vi "IMUCompute.vi"(10 "Cluster":T16 {"navX Device TypeDef"."navX Common Information"."Update Rate (4Hz-60Hz)" min=4 max=50 step=1; "navX Device TypeDef"."navX System Information"."Status"."NAVX_OP_STATUS" items=["INITIALIZING", "SELFTEST_IN_PROGRESS", "ERROR", "IMU_AUTOCAL_IN_PROGRESS", "NORMAL"]; "navX Device TypeDef"."navX System Information"."Status"."NAVX_CAL_STATUS" items=["IMU_CAL_STATE_MASK"=3, "IMU_CAL_INPROGRESS"=0, "IMU_CAL_ACCUMULATE"=1, "IMU_CAL_COMPLETE"=2, "MAG_CAL_COMPLETE"=4, "BARO_CAL_COMPLETE"=8]; "navX Device TypeDef"."navX Interface Protocol TypeDefs"."I2CDevRef"."Device Address" format="%.0x"}) -> ()   [LabVIEW 2014]
uses:
  NavX/roborio/labview/navX-MXP Library/COMMON/TypeDefs/Data TypeDefs/navX Vector Data.ctl
  NavX/roborio/labview/navX-MXP Library/COMMON/TypeDefs/navX Device TypeDef.ctl
  NavX/roborio/labview/navX-MXP Library/COMMON/TypeDefs/Value TypeDefs/navX Interface Protocol.ctl
  <vilib>/Rock Robotics/WPI/SPI/WPI_SPIDevRef.ctl
  <vilib>/Rock Robotics/SystemInterfaces/Typedef/FPGA_TypedefDigitalModule.ctl
  <vilib>/Rock Robotics/SystemInterfaces/spilib/spi_bus.ctl
  <vilib>/Rock Robotics/WPI/I2C/WPI_I2CDevRef.ctl
  <vilib>/Rock Robotics/SystemInterfaces/i2clib/i2c_bus.ctl
  NavX/roborio/labview/navX-MXP Library/COMMON/TypeDefs/Data TypeDefs/navX Board Information.ctl
  NavX/roborio/labview/navX-MXP Library/COMMON/TypeDefs/Data TypeDefs/navX Status Data.ctl
  NavX/roborio/labview/navX-MXP Library/COMMON/TypeDefs/Value TypeDefs/navX NAVX_OP_STATUS.ctl
  NavX/roborio/labview/navX-MXP Library/COMMON/TypeDefs/Value TypeDefs/navX NAVX_CAL_STATUS.ctl
  NavX/roborio/labview/navX-MXP Library/COMMON/TypeDefs/Value TypeDefs/navX NAVX_SENSOR_STATUS.ctl
  NavX/roborio/labview/navX-MXP Library/COMMON/TypeDefs/Data TypeDefs/navX Offsets Data.ctl
  NavX/roborio/labview/navX-MXP Library/COMMON/TypeDefs/Value TypeDefs/navX Update Rate.ctl
  <vilib>/Rock Robotics/Network Tables/SD Write Number.vi
  <vilib>/Rock Robotics/Network Tables/SD Write Numeric Array.vi
  Global 5.vi
  NavX/roborio/labview/navX-MXP Library/navX-MXP IMU.lvlib
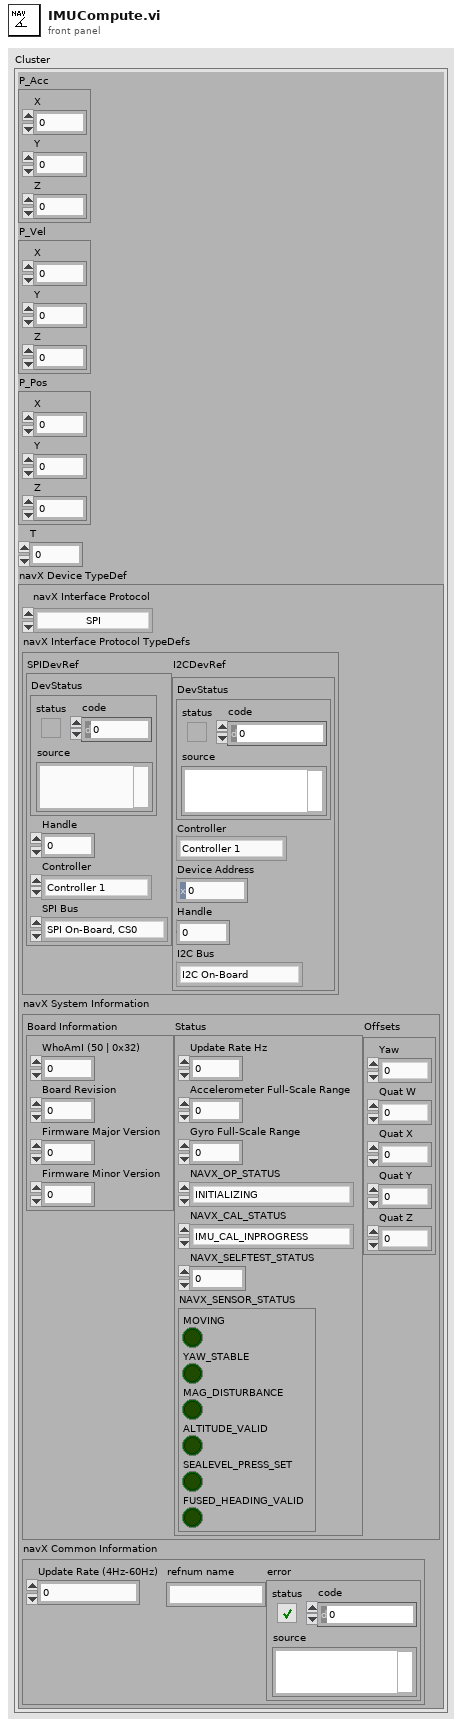
[diagram p1: front panel]
types:
  T1 = typedef "navX-MXP IMU.lvlib/navX Vector Data.ctl" = cluster{"X":dbl, "Y":dbl, "Z":dbl}
  T2 = typedef "navX-MXP IMU.lvlib/navX Device TypeDef.ctl" = cluster{"navX Interface Protocol":T3, "navX Interface Protocol TypeDefs":cluster{"SPIDevRef":T4, "I2CDevRef":T7}, "navX System Information":cluster{"Board Information":T9, "Status":T10, "Offsets":T14}, "navX Common Information":cluster{"Update Rate (4Hz-60Hz)":T15, "refnum name":string, "error":errorcluster}}
  T3 = typedef "navX-MXP IMU.lvlib/navX Interface Protocol.ctl" = enum16{"SPI", "I2C"}
  T4 = typedef "WPI_SPIDevRef.ctl" = cluster{"DevStatus":errorcluster, "Handle":i32, "Controller":T5, "SPI Bus":T6}
  T5 = typedef "FPGA_TypedefDigitalModule.ctl" = enum16{"Controller 1"}
  T6 = typedef "spi_bus.ctl" = enum16{"SPI On-Board, CS0", "SPI On-Board, CS1", "SPI On-Board, CS2", "SPI On-Board, CS3", "SPI MXP", "Invalid"}
  T7 = typedef "WPI_I2CDevRef.ctl" = cluster{"DevStatus":errorcluster, "Controller":T5, "Device Address":u8, "Handle":i32, "I2C Bus":T8}
  T8 = typedef "i2c_bus.ctl" = enum16{"I2C On-Board", "I2C MXP", "Invalid"}
  T9 = typedef "navX-MXP IMU.lvlib/navX Board Information.ctl" = cluster{"WhoAmI (50 | 0x32)":u8, "Board Revision":u8, "Firmware Major Version":u8, "Firmware Minor Version":u8}
  T10 = typedef "navX-MXP IMU.lvlib/navX Status Data.ctl" = cluster{"Update Rate Hz":u8, "Accelerometer Full-Scale Range":u8, "Gyro Full-Scale Range":u16, "NAVX_OP_STATUS":T11, "NAVX_CAL_STATUS":T12, "NAVX_SELFTEST_STATUS":u8, "NAVX_SENSOR_STATUS":T13}
  T11 = typedef "navX-MXP IMU.lvlib/navX NAVX_OP_STATUS.ctl" = u8
  T12 = typedef "navX-MXP IMU.lvlib/navX NAVX_CAL_STATUS.ctl" = u8
  T13 = typedef "navX-MXP IMU.lvlib/navX NAVX_SENSOR_STATUS.ctl" = cluster{"MOVING":bool, "YAW_STABLE":bool, "MAG_DISTURBANCE":bool, "ALTITUDE_VALID":bool, "SEALEVEL_PRESS_SET":bool, "FUSED_HEADING_VALID":bool}
  T14 = typedef "navX-MXP IMU.lvlib/navX Offsets Data.ctl" = cluster{"Yaw":dbl, "Quat W":dbl, "Quat X":dbl, "Quat Y":dbl, "Quat Z":dbl}
  T15 = typedef "navX-MXP IMU.lvlib/navX Update Rate.ctl" = u8
  T16 = cluster{"P_Acc":T1, "P_Vel":T1, "P_Pos":T1, "T":i32, "navX Device TypeDef":T2}
  T17 = typedef "navX-MXP IMU.lvlib/navX Quaternion Data.ctl" = cluster{"W":dbl, "X":dbl, "Y":dbl, "Z":dbl}
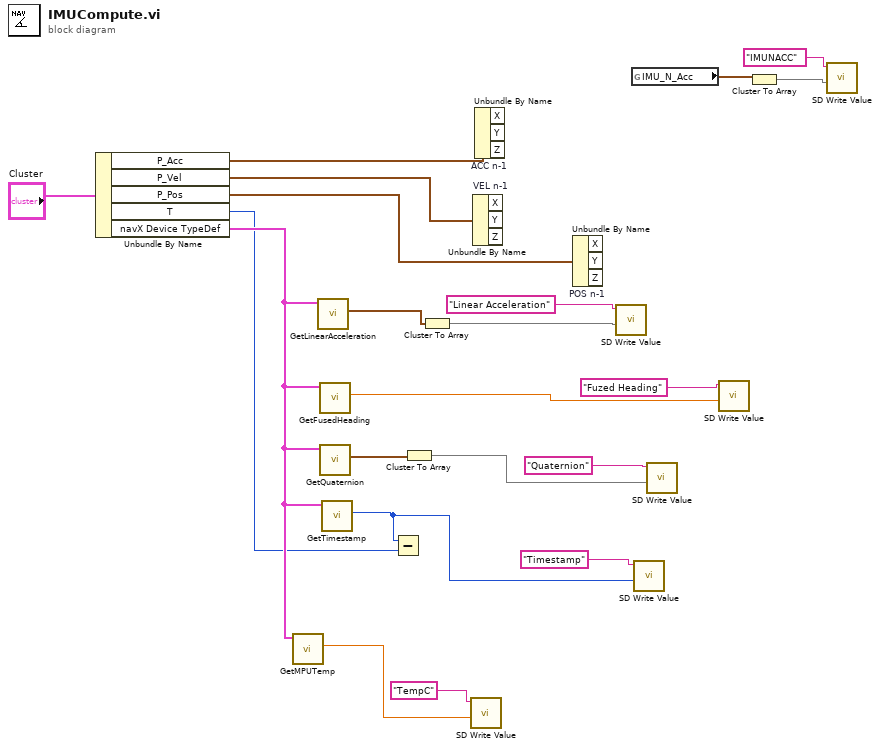
[diagram p0: block diagram]
diagram:
  n1 = Unbundle By Name("Cluster") -> ("P_Acc"=w18:T1, "P_Vel"=w17:T1, "P_Pos"=w16:T1, "T"=w19:i32, "navX Device TypeDef"=w20:T2)
  n2 = call "GetMPUTemp.vi"("navX Device TypeDef"=w20) -> ("MPU Temperature (Centigrade)"=w6:dbl)  [unwired: 8 in, 2 out]
  n3 = call "GetLinearAcceleration.vi"("navX Device TypeDef"=w20) -> ("Linear Acceleration"=w9:T1)  [unwired: 8 in, 2 out]
  n4 = call "GetFusedHeading.vi"("navX Device TypeDef"=w20) -> ("Fused Heading"=w11:dbl)  [unwired: 8 in, 2 out]
  n5 = call "GetQuaternion.vi"("navX Device TypeDef"=w20) -> ("Quaternion"=w14:T17)  [unwired: 8 in, 2 out]
  n6 = call "GetTimestamp.vi"("navX Device TypeDef"=w20) -> ("Timestamp"=w4:u32)  [unwired: 8 in, 2 out]
  n7 = Subtract(x=w4, y=w19) -> ()  [unwired: 1 out]
  n8 = Cluster To Array(cluster=w14) -> (array=w13:dbl[])
  n9 = Cluster To Array(cluster=w9) -> (array=w8:dbl[])
  n10 = call-poly <vilib>:"SD Write Value.vi"("Numeric"=w6, "Name"="TempC") -> ()  [unwired: 8 in, 2 out]
  n11 = Unbundle By Name "VEL n-1"(w17) -> ()  [unwired: 3 out]
  n12 = Unbundle By Name "ACC n-1"(w18) -> ()  [unwired: 3 out]
  n13 = Unbundle By Name "POS n-1"(w16) -> ()  [unwired: 3 out]
  n14 = call-poly <vilib>:"SD Write Value.vi"("Numeric Array"=w8, "Name"="Linear Acceleration") -> ()  [unwired: 8 in, 2 out]
  n15 = global read "Global 5.vi" "IMU_N_Acc"() -> (w3:T1)
  n16 = call-poly <vilib>:"SD Write Value.vi"("Numeric"=w4, "Name"="Timestamp") -> ()  [unwired: 8 in, 2 out]
  n17 = call-poly <vilib>:"SD Write Value.vi"("Numeric Array"=w13, "Name"="Quaternion") -> ()  [unwired: 8 in, 2 out]
  n18 = call-poly <vilib>:"SD Write Value.vi"("Numeric"=w11, "Name"="Fuzed Heading") -> ()  [unwired: 8 in, 2 out]
  n19 = Cluster To Array(cluster=w3) -> (array=w2:dbl[])
  n20 = call-poly <vilib>:"SD Write Value.vi"("Numeric Array"=w2, "Name"="IMUNACC") -> ()  [unwired: 8 in, 2 out]
